vi "catalog.create_dataset.vi"(8 "error in":errorcluster, 10 "name":string, 11 "Nominal Client in":refnum<class "Nominal Client.lvclass">) -> (0 "error out":errorcluster, 2 "Dataset":refnum<class "dataset.lvclass">, 3 "Nominal Client out":refnum<class "Nominal Client.lvclass">)   [LabVIEW 2020, in "Nominal Client.lvclass"]
doc: "<b> UNDER DEVELOPMENT! Do not use function </b>"
uses:
  Nominal Client.lvclass
  datasources/dataset/dataset.lvclass/dataset.ctl
  datasources/dataset/rid.set.vi
  datasources/dataset/datasetName.set.vi
  datasources/dataset/datasetDescription.set.vi
  datasources/dataset/object.set.vi
  <vilib>/JDP Science/JSONtext/JSON text to Variant.vi
  <vilib>/JDP Science/JSONtext/LVClass Serializer/JSONtext LVClass Serializer.lvclass
  Nominal Client.lvclass/Nominal Client.ctl
  datasources/dataset/dataset.lvclass
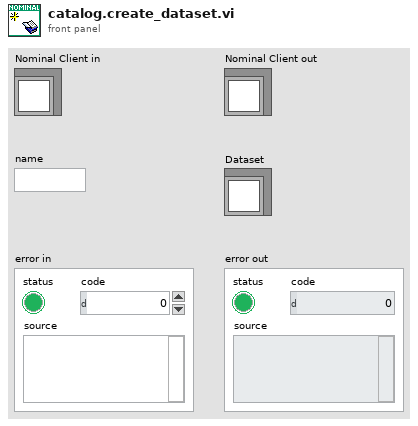
[diagram p1: front panel]
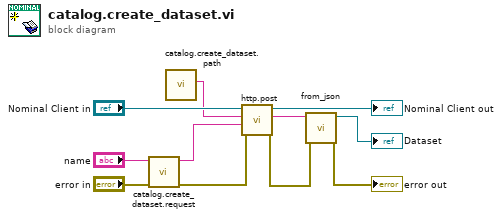
[diagram p0: block diagram]
diagram:
  n1 = call "catalog.create_dataset.request.vi"("error in"="error in", "name"="name") -> ("error out"=w6:errorcluster, "request"=w5:string)  [unwired: 8 in]
  n2 = call "catalog.create_dataset.path.vi"() -> ("path"=w9:string)  [unwired: 11 in]
  n3 = call "http.post.vi"("error in"=w6, "Request body"=w5, "Path"=w9, "Nominal Client in"="Nominal Client in") -> ("error out"=w3:errorcluster, "Response"=w4:string, "Nominal Client out"=→"Nominal Client out":refnum<class "Nominal Client.lvclass">)  [unwired: 4 in, 1 out]
  n4 = call "from_json.vi"("error in"=w3, "dataset JSON"=w4) -> ("error out"=→"error out":errorcluster, "Dataset"=→"Dataset":refnum<class "dataset.lvclass">)  [unwired: 8 in]
